vi "Shutdown.vi"(8 "error in (no error)":errorcluster, 11 "DemoDAQ in":refnum<class "DemoDAQ.lvclass">) -> (0 "error out":errorcluster, 3 "DemoDAQ out":refnum<class "DemoDAQ.lvclass">)   [LabVIEW 2020, in "DemoDAQ.lvlib" / "DemoDAQ.lvclass"]
uses:
  DemoDAQ.lvclass
  Hardware Abstraction Layer/Component/DAQ/DAQ/DAQ.lvclass
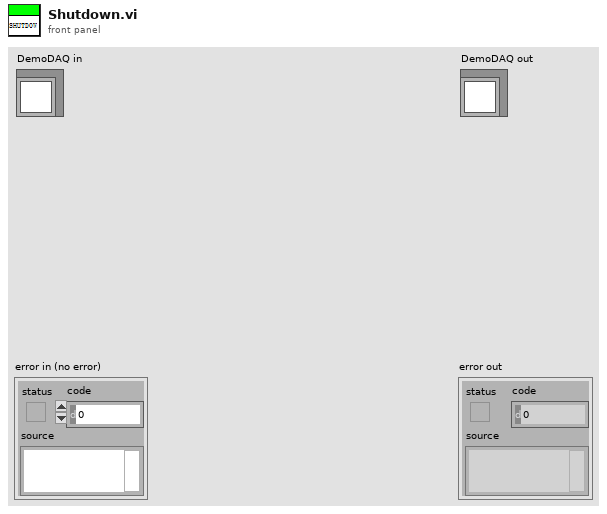
[diagram p1: front panel]
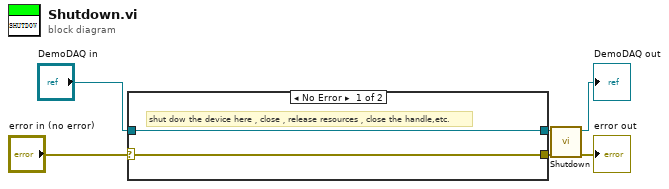
[diagram p0: block diagram]
diagram:
  n1 = case shown="No Error" "error in (no error)" {
    selector: "error in (no error)" -> [w7 w10]
    tunnel: [w7 w10] -> w1
    tunnel: [w8 w9] -> w2
    tunnel: "DemoDAQ in" -> [w8 w9]
    frame No Error {
      # "shut dow the device here，close，release resources，close the handle,etc."
    }
    frame Error {
    }
  }
  n2 = call-parent "Shutdown.vi"("error in (no error)"=w1, "GRMActor in"=w2) -> ("error out"=→"error out":errorcluster, "GRMActor out"=→"DemoDAQ out":refnum<class "DemoDAQ.lvclass">)  [unwired: 8 in]
